vi "Scaling.vi"(8 "error in (no error)":errorcluster, 11 "Group in":refnum<class "Group.lvclass">) -> (0 "error out":errorcluster, 2 "Scaling":refnum<class "Scaling.lvclass">, 3 "Group out":refnum<class "Group.lvclass">)   [LabVIEW 2020, in "VolatusConfig.lvlib" / "Group.lvclass"]
uses:
  Group.lvclass
  Group.lvclass/Group.ctl
  Scaling/Scaling.lvclass
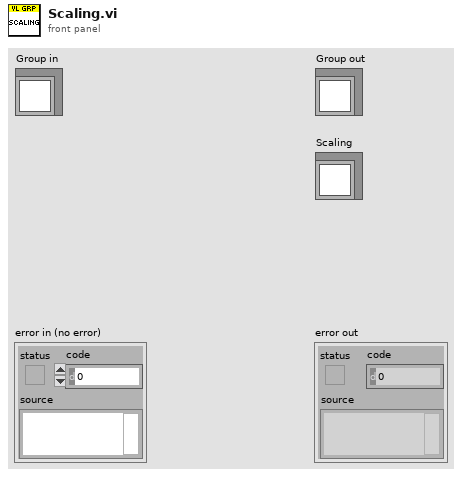
[diagram p1: front panel]
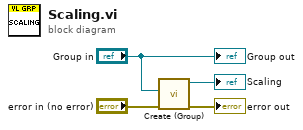
[diagram p0: block diagram]
diagram:
  n1 = call "Create (Group).vi"("error in (no error)"="error in (no error)", "Group Config"="Group in") -> ("error out"=→"error out":errorcluster, "Scaling out"=→"Scaling":refnum<class "Scaling.lvclass">)  [unwired: 8 in]
  "Group out" <- "Group in"
